vi "ascii转文本.vi"(11 "输入":string) -> (2 "错误输出":bool, 3 "输出":string)   [LabVIEW 2018]
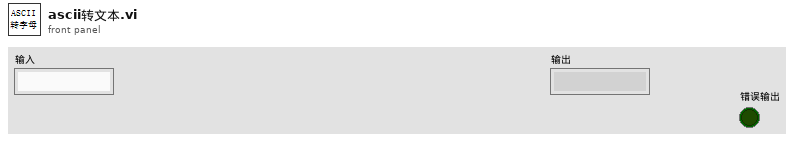
[diagram p1: front panel]
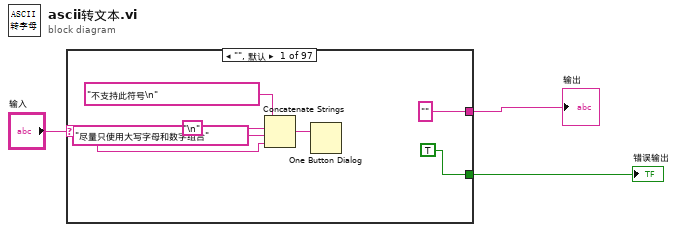
[diagram p0: block diagram]
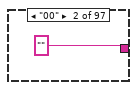
[diagram p2: hidden frame]
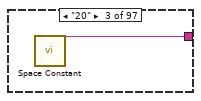
[diagram p3: hidden frame]
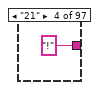
[diagram p4: hidden frame]
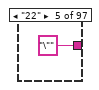
[diagram p5: hidden frame]
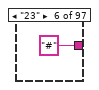
[diagram p6: hidden frame]
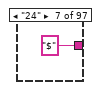
[diagram p7: hidden frame]
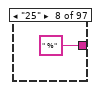
[diagram p8: hidden frame]
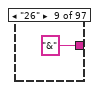
[diagram p9: hidden frame]
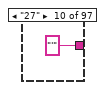
[diagram p10: hidden frame]
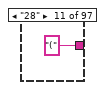
[diagram p11: hidden frame]
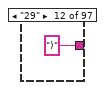
[diagram p12: hidden frame]
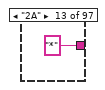
[diagram p13: hidden frame]
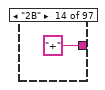
[diagram p14: hidden frame]
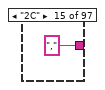
[diagram p15: hidden frame]
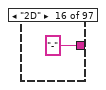
[diagram p16: hidden frame]
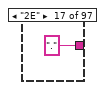
[diagram p17: hidden frame]
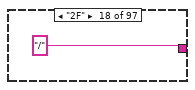
[diagram p18: hidden frame]
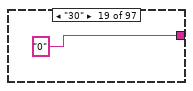
[diagram p19: hidden frame]
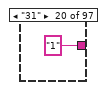
[diagram p20: hidden frame]
diagram:
  n1 = case shown="\"\", 默认" "输入" {
    selector: "输入" -> [w6 _ _ _ _ _ _ _ _ _ _ _ _ _ _ _ _ _ _ _ _ _ _ _ _ _ _ _ _ _ _ _ _ _ _ _ _ _ _ _ _ _ _ _ _ _ _ _ _ _ _ _ _ _ _ _ _ _ _ _ _ _ _ _ _ _ _ _ _ _ _ _ _ _ _ _ _ _ _ _ _ _ _ _ _ _ _ _ _ _ _ _ _ _ _ _ _]
    tunnel: ["" "" w12 "!" "\"" "#" "$" " %" "&" "'" "(" ")" "*" "+" "," "-" "." "/" "0" "1" "2" "3" "4" "5" "6" "7" "8" "9" ":" ("String") ";" ("String") "<" ("String") "=" ("String") ">" ("String") "\t?" ("String") "@" "A" "B" "C" "D" "E" "F" "G" "H" "I" "J" "K" "L" "M" "N" "O" "P" "Q" "R" "S" "T" "U" "V" "W" "X" "Y" "Z" "\t[" ("String") "\\" ("String") "]" ("String") "^" ("String") "_\t" ("String") "`" "a" "b" "c" "d" "e" "f" "g" "h" "i" "j" "k" "l" "m" "n" "o" "p" "q" "r" "s" "t" "u" "v" "w" "x" "y" "z" "{" "|" ("String") "}" ("String") "\t~" ("String")] -> w3
    tunnel: [TRUE _ _ _ _ _ _ _ _ _ _ _ _ _ _ _ _ _ _ _ _ _ _ _ _ _ _ _ _ _ _ _ _ _ _ _ _ _ _ _ _ _ _ _ _ _ _ _ _ _ _ _ _ _ _ _ _ _ _ _ _ _ _ _ _ _ _ _ _ _ _ _ _ _ _ _ _ _ _ _ _ _ _ _ _ _ _ _ _ _ _ _ _ _ _ _ _] -> w1
    frame "", Default {
      n2 = Concatenate Strings("不支持此符号\n" ("消息"), "\n", "尽量只使用大写字母和数字组合" ("字符串"), w6) -> (w5:string)
      n3 = One Button Dialog(message=w5) -> ()  [unwired: 1 in, 1 out]
    }
    frame "00" {
    }
    frame "20" {
      n4 = call <vilib>:"Space Constant.vi"() -> ("String"=w12:string)
    }
    frame "21" {
    }
    frame "22" {
    }
    frame "23" {
    }
    frame "24" {
    }
    frame "25" {
    }
    frame "26" {
    }
    frame "27" {
    }
    frame "28" {
    }
    frame "29" {
    }
    frame "2A" {
    }
    frame "2B" {
    }
    frame "2C" {
    }
    frame "2D" {
    }
    frame "2E" {
    }
    frame "2F" {
    }
    frame "30" {
    }
    frame "31" {
    }
    frame "32" {
    }
    frame "33" {
    }
    frame "34" {
    }
    frame "35" {
    }
    frame "36" {
    }
    frame "37" {
    }
    frame "38" {
    }
    frame "39" {
    }
    frame "3A" {
    }
    frame "3B" {
    }
    frame "3C" {
    }
    frame "3D" {
    }
    frame "3E" {
    }
    frame "3F" {
    }
    frame "40" {
    }
    frame "41" {
    }
    frame "42" {
    }
    frame "43" {
    }
    frame "44" {
    }
    frame "45" {
    }
    frame "46" {
    }
    frame "47" {
    }
    frame "48" {
    }
    frame "49" {
    }
    frame "4A" {
    }
    frame "4B" {
    }
    frame "4C" {
    }
    frame "4D" {
    }
    frame "4E" {
    }
    frame "4F" {
    }
    frame "50" {
    }
    frame "51" {
    }
    frame "52" {
    }
    frame "53" {
    }
    frame "54" {
    }
    frame "55" {
    }
    frame "56" {
    }
    frame "57" {
    }
    frame "58" {
    }
    frame "59" {
    }
    frame "5A" {
    }
    frame "5B" {
    }
    frame "5C" {
    }
    frame "5D" {
    }
    frame "5E" {
    }
    frame "5F" {
    }
    frame "60" {
    }
    frame "61" {
    }
    frame "62" {
    }
    frame "63" {
    }
    frame "64" {
    }
    frame "65" {
    }
    frame "66" {
    }
    frame "67" {
    }
    frame "68" {
    }
    frame "69" {
    }
    frame "6A" {
    }
    frame "6B" {
    }
    frame "6C" {
    }
    frame "6D" {
    }
    frame "6E" {
    }
    frame "6F" {
    }
    frame "70" {
    }
    frame "71" {
    }
    frame "72" {
    }
    frame "73" {
    }
    frame "74" {
    }
    frame "75" {
    }
    frame "76" {
    }
    frame "77" {
    }
    frame "78" {
    }
    frame "79" {
    }
    frame "7A" {
    }
    frame "7B" {
    }
    frame "7C" {
    }
    frame "7D" {
    }
    frame "7E" {
    }
  }
  "输出" <- w3
  "错误输出" <- w1
